vi "QueueMidi2.vi"() -> ()   [LabVIEW 2014]
uses:
  Controls/MidiCommand.ctl
panel:
  out "Queue Out":u8[](array[numeric]) format="%08b"
  out "Byte From Read":u8[](array[numeric]) format="%08b"
  out "# elements in queue":i32
  out "Commands":T1[](array[typedef])
  out "Messages Queued":i32
  out "Timeouts Occured":i32
  in  "Queue Name":string="Midi In"
  in  "Timeout (ms)\n(-1: None)":i32=1000
  in  "Character Count":u32=1
  in  "stop":bool
  in  "error in (no error)":errorcluster
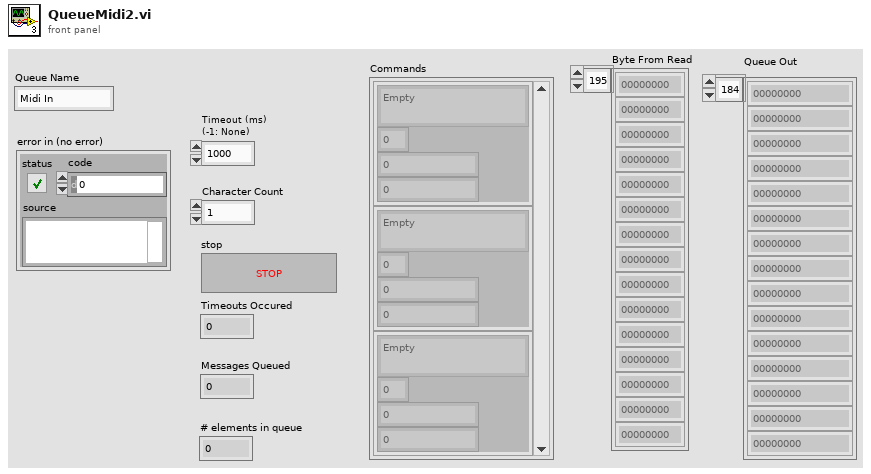
[diagram p1: front panel]
types:
  T1 = typedef "MidiCommand.ctl" = cluster{"Function":enum16{"Empty", "Note Off", "Note On", "Polyphonic Aftertouch", "Control/Mode Change", "Program Change", "Channel Aftertouch", "Pitch Bend Change", "System"}, "Channel":u8, "Data Byte 1":u8, "Data Byte 2":u8}
  T2 = cluster{"Invert Polarity?":bool, "baud rate (9600)":u32, "data bits (8)":u16, "parity (0:none)":u16, "stop bits (10: 1 bit)":u16}
  T3 = enum16{"Empty", "Note Off", "Note On", "Polyphonic Aftertouch", "Control/Mode Change", "Program Change", "Channel Aftertouch", "Pitch Bend Change", "System"}
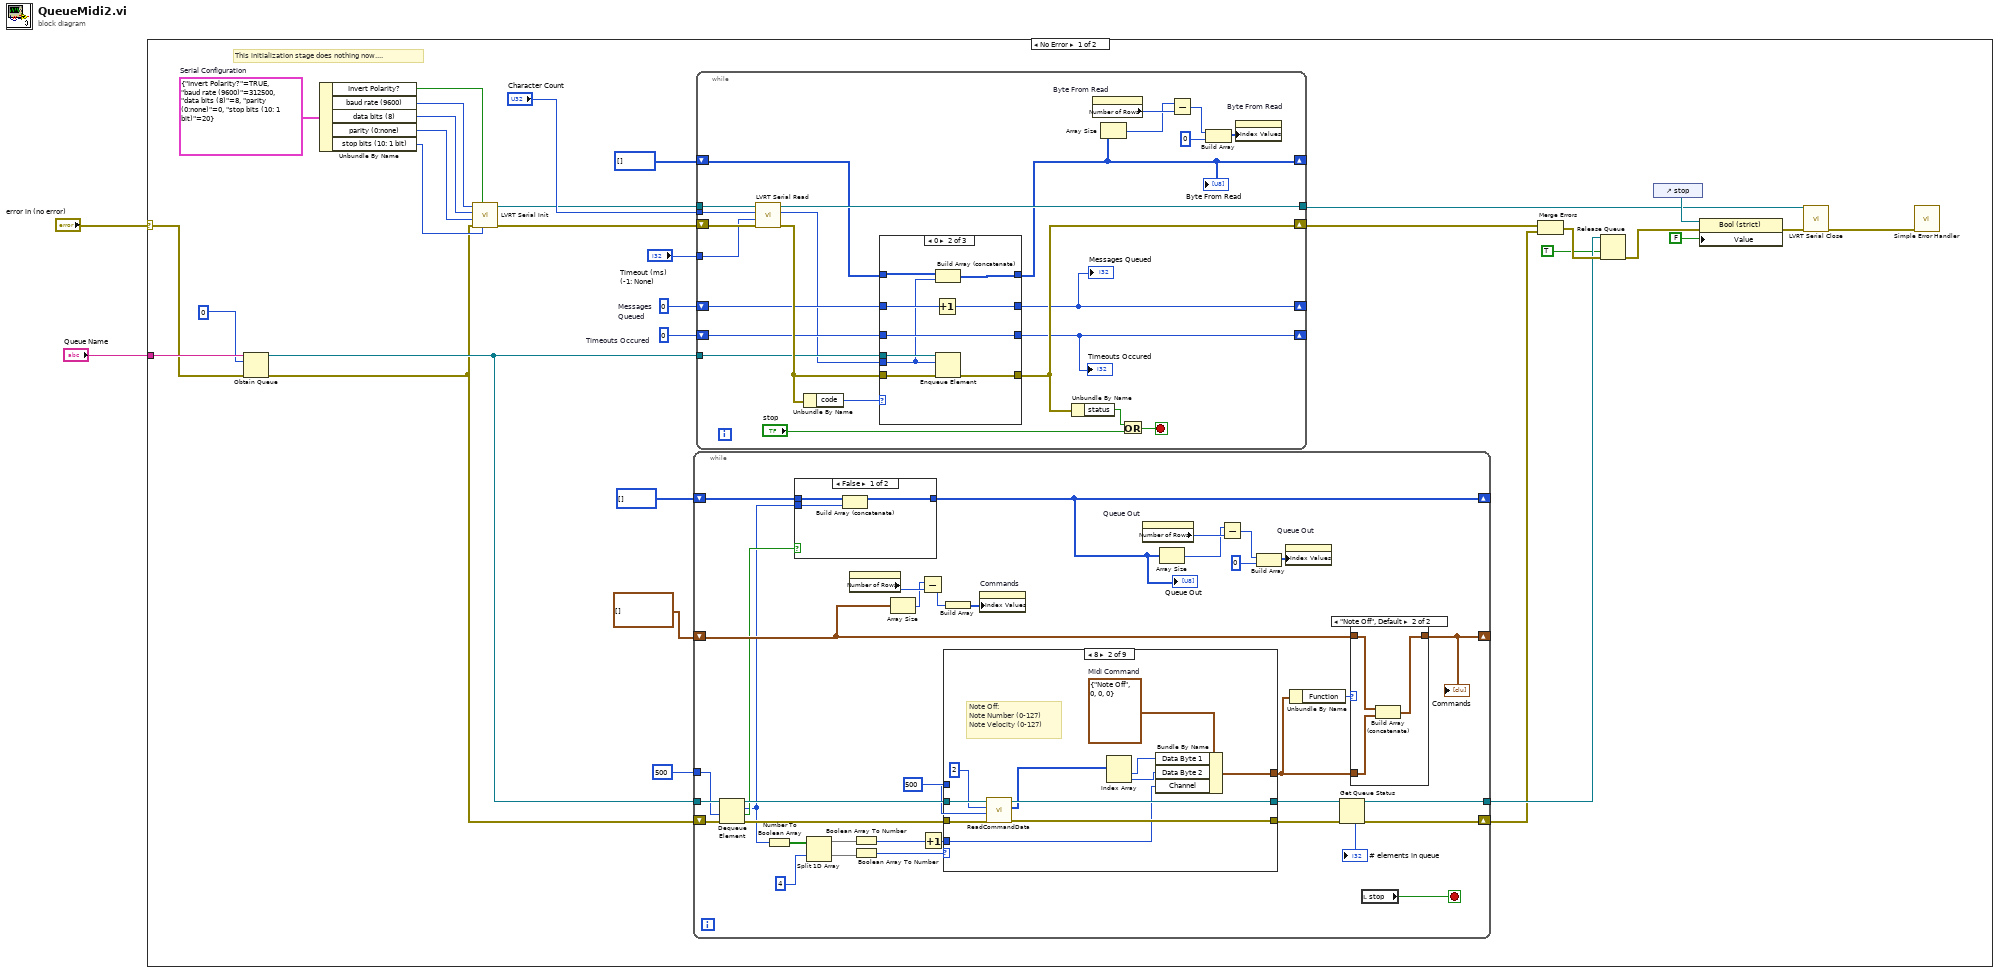
[diagram p0: block diagram]
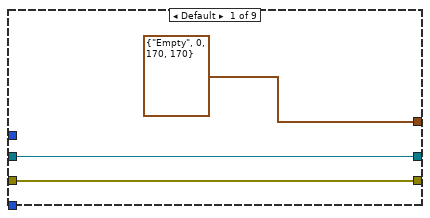
[diagram p4: hidden frame]
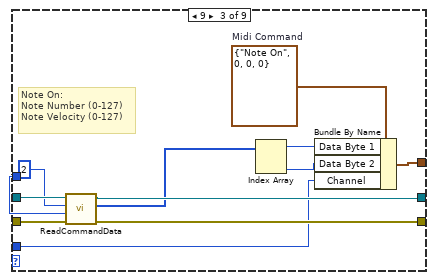
[diagram p5: hidden frame]
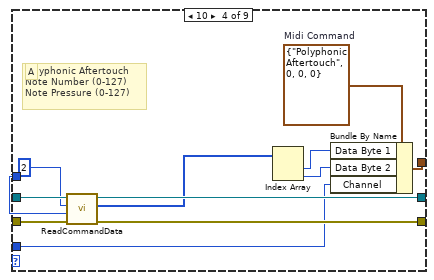
[diagram p6: hidden frame]
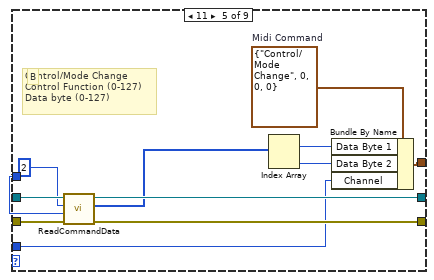
[diagram p7: hidden frame]
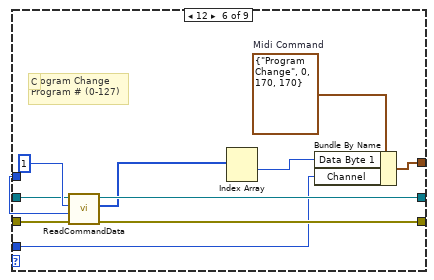
[diagram p8: hidden frame]
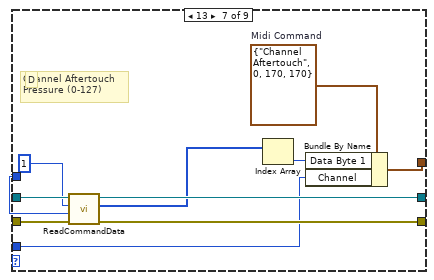
[diagram p9: hidden frame]
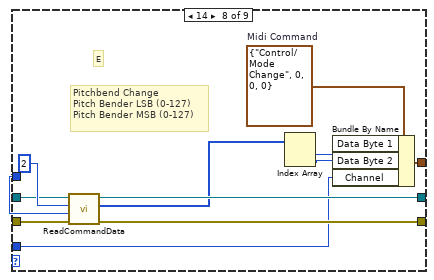
[diagram p10: hidden frame]
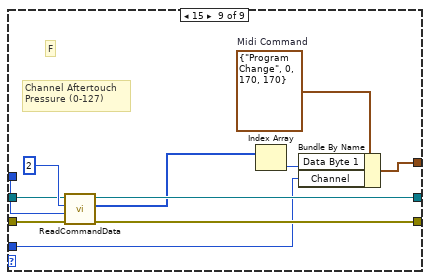
[diagram p11: hidden frame]
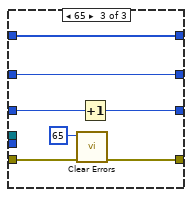
[diagram p13: hidden frame]
diagram:
  n1 = case shown="No Error" "error in (no error)" {
    selector: "error in (no error)" -> [w23 _]
    tunnel: "Queue Name" -> [w24 _]
    frame No Error {
      w21 = 0  # Messages Queued
      w22 = 0  # Timeouts Occured
      w34 = T2 {"Invert Polarity?"=TRUE, "baud rate (9600)"=312500, "data bits (8)"=8, "parity (0:none)"=0, "stop bits (10: 1 bit)"=20}  # Serial Configuration
      # "This initialization stage does nothing now...."
      n2 = Obtain Queue(name (unnamed)=w24, element data type=u8 0, error in (no error)=w23) -> (queue out=w20:refnum<queue>, error out=w18:errorcluster)  [unwired: 2 in, 1 out]
      n3 = Unbundle By Name(w34) -> ("Invert Polarity?"=w28:bool, "baud rate (9600)"=w32:u32, "data bits (8)"=w31:u16, "parity (0:none)"=w30:u16, "stop bits (10: 1 bit)"=w29:u16)
      n4 = call "LVRT Serial Init.vi"("stop bits (10: 1 bit)"=w29, "Invert Polarity?"=w28, "error in (no error)"=w18, "parity (0:none)"=w30, "data bits (8)"=w31, "baud rate (9600)"=w32) -> ("error out"=w26:errorcluster, "FPGA Main Reference Out"=w27:refnum<k20>)  [unwired: 4 in]
      n5 = while {
        tunnel: w20 -> [w70]
        shift-right: [w61] -> w7
        shift-left: w18 -> [w67]
        shift-right: [w64] -> _
        shift-left: T1[] [] -> [w56]
        tunnel: [w58] -> w8
        shift-right: [w42] -> _
        shift-left: u8[] [] -> [w50]
        tunnel: 500 ("timeout in ms (-1)") -> [w45]
        stop <- w69 stop-if-true
        n6 = Dequeue Element(queue=w70, timeout in ms (-1)=w45, error in (no error)=w67) -> (queue out=w65:refnum<queue>, element=w35:u8, timed out?=w51:bool, error out=w66:errorcluster)
        n7 = Number To Boolean Array(number=w35) -> (Boolean array=w40:bool[])
        n8 = case shown="False" w51 {
          tunnel: w50 -> [w73 w74]
          tunnel: w35 -> [w72 _]
          tunnel: [w71 w74] -> w42
          frame False {
            n9 = Build Array (concatenate)(w73, w72) -> (w71:u8[])
          }
          frame True {
          }
        }
        "Queue Out" <- w42
        n10 = Split 1D Array(array=w40, index=4) -> (first subarray=w38:bool[], second subarray=w39:bool[])
        n11 = property on="Commands" class="Arr (strict)"() -> ("Number of Rows"=w54:u32)  [unwired: 2 in, 2 out]
        n12 = Boolean Array To Number(Boolean array=w38) -> (number=w36:u32)
        n13 = Boolean Array To Number(Boolean array=w39) -> (number=w37:u32)
        n14 = Array Size(array=w56) -> (size(s)=w53:i32)
        n15 = Subtract(x=w53, y=w54) -> (x-y=w52:u32)
        n16 = Increment(x=w36) -> (x+1=w44:u32)
        n17 = case shown="8" w37 {
          tunnel: [w80 w92 w102 w114 w127 w138 w149 w161 w173] -> w59
          tunnel: [w81 w84 w105 w116 w128 w139 w150 w162 w174] -> w60
          tunnel: w66 -> [w81 w93 w104 w117 w129 w140 w151 w163 w172]
          tunnel: w65 -> [w80 w91 w103 w115 w126 w136 w148 w159 w170]
          tunnel: 500 ("timeout in ms (-1)") -> [_ w89 w100 w112 w124 w135 w146 w158 w169]
          tunnel: [T1 {"Function"=enum."Empty", "Channel"=0, "Data Byte 1"=170, "Data Byte 2"=170} ("Midi Command") w87 w97 w110 w121 w133 w143 w155 w166] -> w63
          tunnel: w44 -> [_ w82 w94 w106 w119 w132 w141 w154 w164]
          frame Default {
          }
          frame 8 {
            w88 = T1 {"Function"=enum."Note Off", "Channel"=0, "Data Byte 1"=0, "Data Byte 2"=0}  # Midi Command
            # "Note Off: \nNote Number (0-127)\nNote Velocity (0-127)"
            n18 = call "ReadCommandData.vi"("error in (no error)"=w93, "timeout in ms (-1)"=w89, "Messages To Read"=u32 2, "Queue in"=w91) -> ("error out"=w84:errorcluster, "Data Bytes"=w83:u8[], "Queue in 2"=w92:refnum<queue>)  [unwired: 5 in]
            n19 = Index Array(array=w83) -> (element #1=w86:u8, element #2=w85:u8)  [unwired: 2 in]
            n20 = Bundle By Name(cluster=w88, "Data Byte 1"=w86, "Data Byte 2"=w85, "Channel"=w82) -> (w87:T1)
          }
          frame 9 {
            w98 = T1 {"Function"=enum."Note On", "Channel"=0, "Data Byte 1"=0, "Data Byte 2"=0}  # Midi Command
            # "Note On: \nNote Number (0-127)\nNote Velocity (0-127)"
            n21 = call "ReadCommandData.vi"("error in (no error)"=w104, "timeout in ms (-1)"=w100, "Messages To Read"=u32 2 ("byte count"), "Queue in"=w103) -> ("error out"=w105:errorcluster, "Data Bytes"=w95:u8[], "Queue in 2"=w102:refnum<queue>)  [unwired: 5 in]
            n22 = Index Array(array=w95) -> (element #1=w99:u8, element #2=w96:u8)  [unwired: 2 in]
            n23 = Bundle By Name(cluster=w98, "Data Byte 1"=w99, "Data Byte 2"=w96, "Channel"=w94) -> (w97:T1)
          }
          frame 10 {
            w111 = T1 {"Function"=enum."Polyphonic Aftertouch", "Channel"=0, "Data Byte 1"=0, "Data Byte 2"=0}  # Midi Command
            # "A"
            # "Polyphonic Aftertouch\nNote Number (0-127)\nNote Pressure (0-127)"
            n24 = call "ReadCommandData.vi"("error in (no error)"=w117, "timeout in ms (-1)"=w112, "Messages To Read"=u32 2 ("byte count"), "Queue in"=w115) -> ("error out"=w116:errorcluster, "Data Bytes"=w107:u8[], "Queue in 2"=w114:refnum<queue>)  [unwired: 5 in]
            n25 = Index Array(array=w107) -> (element #1=w109:u8, element #2=w108:u8)  [unwired: 2 in]
            n26 = Bundle By Name(cluster=w111, "Data Byte 1"=w109, "Data Byte 2"=w108, "Channel"=w106) -> (w110:T1)
          }
          frame 11 {
            w123 = T1 {"Function"=enum."Control/Mode Change", "Channel"=0, "Data Byte 1"=0, "Data Byte 2"=0}  # Midi Command
            # "B"
            # "Control/Mode Change\nControl Function (0-127)\nData byte (0-127)"
            n27 = call "ReadCommandData.vi"("error in (no error)"=w129, "timeout in ms (-1)"=w124, "Messages To Read"=u32 2 ("byte count"), "Queue in"=w126) -> ("error out"=w128:errorcluster, "Data Bytes"=w118:u8[], "Queue in 2"=w127:refnum<queue>)  [unwired: 5 in]
            n28 = Index Array(array=w118) -> (element #1=w122:u8, element #2=w120:u8)  [unwired: 2 in]
            n29 = Bundle By Name(cluster=w123, "Data Byte 1"=w122, "Data Byte 2"=w120, "Channel"=w119) -> (w121:T1)
          }
          frame 12 {
            w134 = T1 {"Function"=enum."Program Change", "Channel"=0, "Data Byte 1"=170, "Data Byte 2"=170}  # Midi Command
            # "C"
            # "Program Change\nProgram # (0-127)"
            n30 = call "ReadCommandData.vi"("error in (no error)"=w140, "timeout in ms (-1)"=w135, "Messages To Read"=u32 1 ("byte count"), "Queue in"=w136) -> ("error out"=w139:errorcluster, "Data Bytes"=w130:u8[], "Queue in 2"=w138:refnum<queue>)  [unwired: 5 in]
            n31 = Index Array(array=w130) -> (element #1=w131:u8)  [unwired: 2 in, 1 out]
            n32 = Bundle By Name(cluster=w134, "Data Byte 1"=w131, "Channel"=w132) -> (w133:T1)
          }
          frame 13 {
            w144 = T1 {"Function"=enum."Channel Aftertouch", "Channel"=0, "Data Byte 1"=170, "Data Byte 2"=170}  # Midi Command
            # "Channel Aftertouch\nPressure (0-127)"
            # "D"
            n33 = call "ReadCommandData.vi"("error in (no error)"=w151, "timeout in ms (-1)"=w146, "Messages To Read"=u32 1 ("byte count"), "Queue in"=w148) -> ("error out"=w150:errorcluster, "Data Bytes"=w142:u8[], "Queue in 2"=w149:refnum<queue>)  [unwired: 5 in]
            n34 = Index Array(array=w142) -> (element=w145:u8)  [unwired: 1 in]
            n35 = Bundle By Name(cluster=w144, "Data Byte 1"=w145, "Channel"=w141) -> (w143:T1)
          }
          frame 14 {
            w157 = T1 {"Function"=enum."Control/Mode Change", "Channel"=0, "Data Byte 1"=0, "Data Byte 2"=0}  # Midi Command
            # "E"
            # "Pitchbend Change\nPitch Bender LSB (0-127)\nPitch Bender MSB (0-127)"
            n36 = call "ReadCommandData.vi"("error in (no error)"=w163, "timeout in ms (-1)"=w158, "Messages To Read"=u32 2 ("byte count"), "Queue in"=w159) -> ("error out"=w162:errorcluster, "Data Bytes"=w152:u8[], "Queue in 2"=w161:refnum<queue>)  [unwired: 5 in]
            n37 = Index Array(array=w152) -> (element #1=w156:u8, element #2=w153:u8)  [unwired: 2 in]
            n38 = Bundle By Name(cluster=w157, "Data Byte 1"=w156, "Data Byte 2"=w153, "Channel"=w154) -> (w155:T1)
          }
          frame 15 {
            w168 = T1 {"Function"=enum."Program Change", "Channel"=0, "Data Byte 1"=170, "Data Byte 2"=170}  # Midi Command
            # "F"
            # "Channel Aftertouch\nPressure (0-127)"
            n39 = call "ReadCommandData.vi"("error in (no error)"=w172, "timeout in ms (-1)"=w169, "Messages To Read"=u32 2 ("byte count"), "Queue in"=w170) -> ("error out"=w174:errorcluster, "Data Bytes"=w165:u8[], "Queue in 2"=w173:refnum<queue>)  [unwired: 5 in]
            n40 = Index Array(array=w165) -> (element=w167:u8)  [unwired: 1 in]
            n41 = Bundle By Name(cluster=w168, "Data Byte 1"=w167, "Channel"=w164) -> (w166:T1)
          }
        }
        n42 = Build Array(w52) -> (w55:u32[])
        n43 = property on="Commands" class="Arr (strict)"("Index Values"=w55) -> ()  [unwired: 2 in, 2 out]
        n44 = property on="Queue Out" class="Arr (strict)"() -> ("Number of Rows"=w47:u32)  [unwired: 2 in, 2 out]
        n45 = Array Size(array=w42) -> (size(s)=w43:i32)
        n46 = Subtract(x=w43, y=w47) -> (x-y=w46:u32)
        n47 = Build Array(w46, 0 ("element")) -> (w49:u32[])
        n48 = property on="Queue Out" class="Arr (strict)"("Index Values"=w49) -> ()  [unwired: 2 in, 2 out]
        n49 = Unbundle By Name(w63) -> ("Function"=w62:T3)
        n50 = Get Queue Status(queue=w59, error in (no error)=w60) -> (queue out=w58:refnum<queue>, error out=w61:errorcluster, # elements in queue=→"# elements in queue":i32)  [unwired: 1 in, 5 out]
        n51 = case shown="\"Note Off\", Default" w62 {
          tunnel: w56 -> [w75 w78]
          tunnel: w63 -> [_ w77]
          tunnel: [w75 w76] -> w64
          frame "Empty" {
          }
          frame "Note Off", Default {
            n52 = Build Array (concatenate)(w78, w77) -> (w76:T1[])
          }
        }
        "Commands" <- w64
        n53 = local read "stop"() -> (w69:bool)
      }
      n54 = while {
        shift-right: [w186] -> w14
        shift-left: w26 -> [w193]
        tunnel: "Character Count" -> [w194]
        tunnel: w27 -> [w195]
        tunnel: [w192] -> w11
        tunnel: "Timeout (ms)\n(-1: None)" -> [w191]
        tunnel: w20 -> [w188]
        shift-right: [w185] -> _
        shift-left: w22 -> [w187]
        shift-right: [w183] -> _
        shift-left: w21 -> [w184]
        shift-right: [w177] -> _
        shift-left: u8[] [] -> [w178]
        stop <- w198 stop-if-true
        n55 = call "LVRT Serial Read.vi"("error in (no error)"=w193, "Timeout (ms) (-1: no timeout)"=w191, "Bytes to Read"=w194, "FPGA Main Ref"=w195) -> ("error out"=w189:errorcluster, "Read: Char"=w175:u8, "FPGA Main Ref Out"=w192:refnum<k20>)  [unwired: 5 out]
        n56 = Unbundle By Name(w189) -> ("code"=w190:i32)
        n57 = case shown="0" w190 {
          tunnel: w189 -> [w202 w210 w218]
          tunnel: w188 -> [_ w211 _]
          tunnel: [w202 w209 w217] -> w186
          tunnel: w187 -> [w201 w208 w215]
          tunnel: [w201 w208 w214] -> w185
          tunnel: w184 -> [w200 w207 w213]
          tunnel: [w200 w206 w213] -> w183
          tunnel: [w199 w204 w212] -> w177
          tunnel: w178 -> [w199 w205 w212]
          tunnel: w175 -> [_ w203 _]
          frame 1, Default {
          }
          frame 0 {
            n58 = Increment(x=w207) -> (x+1=w206:i32)
            n59 = Build Array (concatenate)(w205, w203) -> (w204:u8[])
            n60 = Enqueue Element(queue=w211, element=w203, error in (no error)=w210) -> (error out=w209:errorcluster)  [unwired: 1 in, 2 out]
          }
          frame 65 {
            n61 = call <vilib>:"Clear Errors.vi"("error in (no error)"=w218, "specific error code to clear (0: all)"=65) -> ("error out"=w217:errorcluster)  [unwired: 4 in, 1 out]
            n62 = Increment(x=w215) -> (x+1=w214:i32)
          }
        }
        "Timeouts Occured" <- w185
        "Messages Queued" <- w183
        "Byte From Read" <- w177
        n63 = Unbundle By Name(w186) -> ("status"=w197:bool)
        n64 = property on="Byte From Read" class="Arr (strict)"() -> ("Number of Rows"=w180:u32)  [unwired: 2 in, 2 out]
        n65 = Array Size(array=w177) -> (size(s)=w176:i32)
        n66 = Or(x=w197, y="stop") -> (x .or. y?=w198:bool)
        n67 = Subtract(x=w176, y=w180) -> (x-y=w179:u32)
        n68 = Build Array(w179, 0 ("element")) -> (w182:u32[])
        n69 = property on="Byte From Read" class="Arr (strict)"("Index Values"=w182) -> ()  [unwired: 2 in, 2 out]
      }
      n70 = Merge Errors(w14, w7) -> (w10:errorcluster)
      n71 = Release Queue(queue=w8, force destroy? (F)=TRUE, error in (no error)=w10) -> (error out=w9:errorcluster)  [unwired: 2 out]
      n72 = control-ref of="stop"() -> (w16:refnum<vi>)
      n73 = property class="Bool (strict)"(reference=w16, error in=w9, "Value"=FALSE) -> (error out=w13:errorcluster)  [unwired: 1 out]
      n74 = call "LVRT Serial Close.vi"("error out"=w13, "FPGA Main Ref"=w11) -> ("error out"=w12:errorcluster)  [unwired: 9 in]
      n75 = call <vilib>:"Simple Error Handler.vi"("error in (no error)"=w12) -> ()  [unwired: 4 in, 5 out]
    }
    frame Error {
    }
  }
